vi "Send Command.vi"(0 "RefNum in":refnum<vi>, 5 "Active Device Basic Properties":string[][](array[string]), 7 "> Cmd to send >":string, 9 ">Active Device Name >":string, 11 "List of last 10 Commands":string[](array[string])) -> (4 "device fast\nresponse":string, 6 "> last cmd accepted? >":bool, 10 "> latest Expected Slow Response >":string, 15 "List of last 10 Commands out":string[](array[string]))   [LabVIEW 2020]
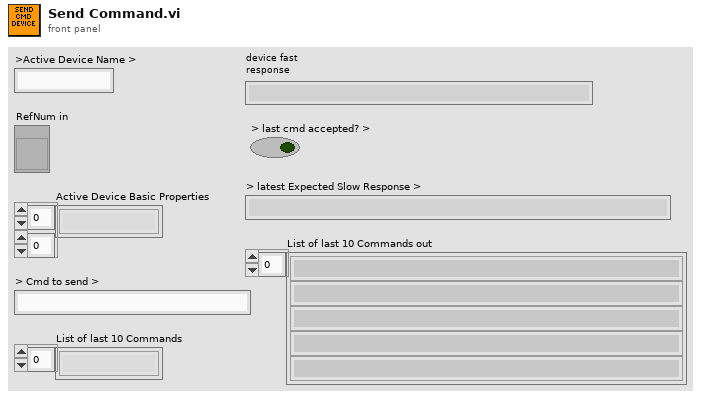
[diagram p1: front panel]
types:
  T1 = typedef "UDP send cluster.ctl" = cluster{"IP Address":string, "UDP Port":string, "Command to Send":string}
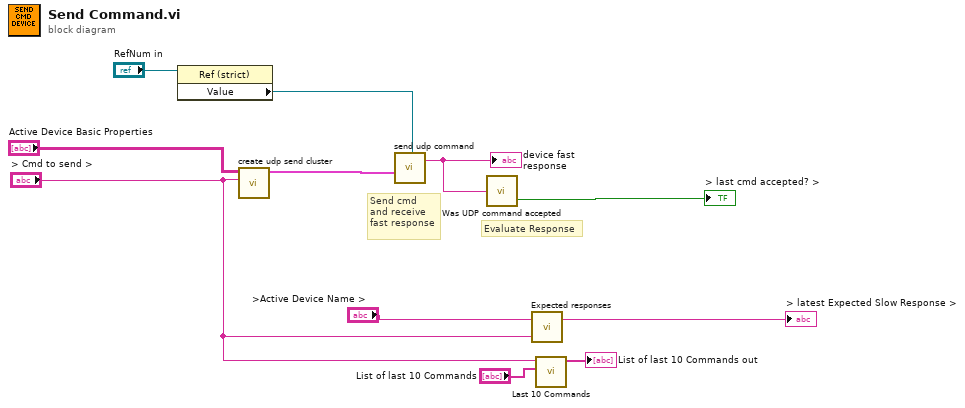
[diagram p0: block diagram]
diagram:
  # "Evaluate Response"
  # "Send cmd\nand receive \nfast response"
  n1 = property class="Ref (strict)"(reference="RefNum in") -> ("Value"=w2:refnum<k16>)  [unwired: 1 in, 2 out]
  n2 = call "create udp send cluster.vi"("Command to send"="> Cmd to send >", "Device Basic Properties"="Active Device Basic Properties") -> ("UDP Send Cluster"=w5:T1)  [unwired: 9 in]
  n3 = call "send udp command.vi"("UDP Send Cluster"=w5, "UDP ID Fast"=w2) -> ("data out"=w6:string)  [unwired: 3 in]
  "device fast\nresponse" <- w6
  n4 = call "Was UDP command accepted.vi"("Fast response"=w6) -> ("Boolean"=→"> last cmd accepted? >":bool)  [unwired: 1 out]
  n5 = call "Expected responses.vi"("Command to Send"="> Cmd to send >", "Device name"=">Active Device Name >") -> ("Expected slow response"=→"> latest Expected Slow Response >":string)  [unwired: 1 out]
  n6 = call "Last 10 Commands.vi"("List of last 10 Commands in"="List of last 10 Commands", "Command to Send"="> Cmd to send >") -> ("List of last 10 Commands out"=→"List of last 10 Commands out":string[])  [unwired: 9 in]
